vi "Header Footer Transform Header Footer [ ].vi"(7 "Header or Footer [ ]":T11[](array[typedef]), 11 "error in (no error)":errorcluster) -> (8 "Header or Footer Complete Cluster":T1, 15 "error out":errorcluster)   [LabVIEW 2012]
doc: "Version 1.0\nDeveloped by Jean-Marc Simard\nCopyright © 2010, Exaprom Inc.\nAll rights reserved.\nLicense: BSD\n\nWith iTextSharp 4.1.6 (http://itextsharp.sourceforge.net)\nunder Mozilla Public License Version 1.1\n(http://www.mozilla.org/MPL/MPL-1.1.html)"
uses:
  Controls/Header Footer cluster.ctl
  Controls/Header Footer Type.ctl
  Controls/Header footer horiz alignment.ctl
  Controls/Cell Vertical alignment.ctl
  Controls/Page number.ctl
  Controls/Font cluster.ctl
  Controls/Font size.ctl
  Controls/Font color.ctl
  C:/Users/MaxCorp/Documents/TopPerm - Base/DLL/itextsharp.dll
  DLL/itextsharp.dll
  Controls/Header Footer Line.ctl
  Controls/Header Footer Complete Cluster.ctl
  Controls/Header Footer Cluster with references.ctl
panel:
  # "X"
  # "Y"
  # "X"
  # "Y"
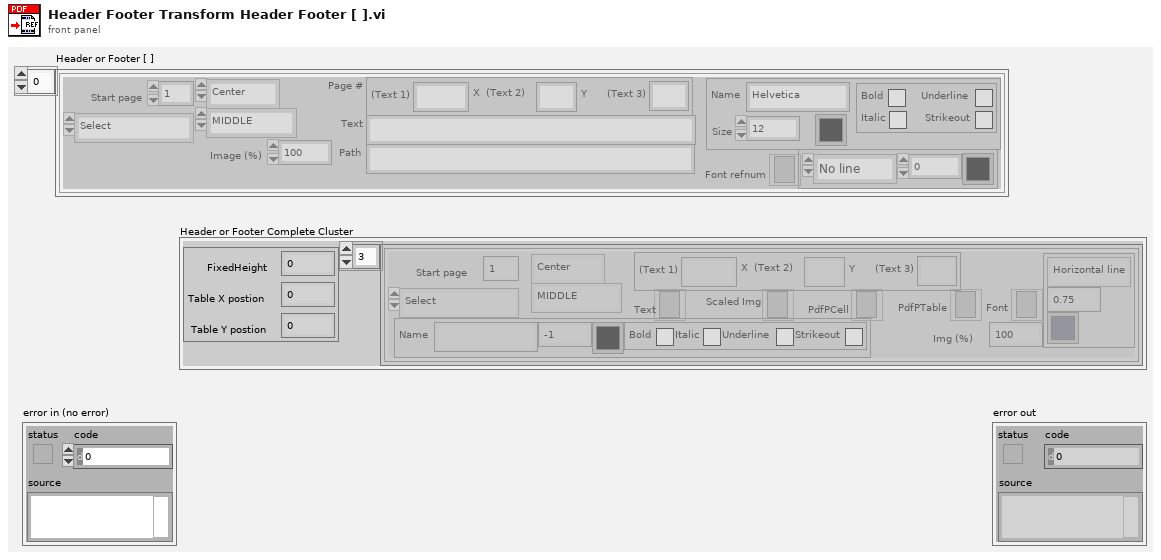
[diagram p1: front panel]
types:
  T1 = typedef "Header Footer Complete Cluster.ctl" = cluster{"Table position":cluster{"FixedHeight":dbl, "Table X postion":dbl, "Table Y postion":dbl}, "Header Footer Cluster with references [ ]":T2[]}
  T2 = typedef "Header Footer Cluster with references.ctl" = cluster{"Start page":i32, "Type":T3, "Alignment":T4, "Vertical Alignement":T5, "Page #":T6, "Text":refnum<k24>, "Scaled Img":refnum<k24>, "PdfPCell":refnum<k24>, "PdfPTable":refnum<k24>, "Font Cluster":T7, "Font ":refnum<k24>, "Img (%)":sgl, "Line":cluster{"Line":T10, "Thickness (points)":sgl, "Colour":T9}}
  T3 = typedef "Header Footer Type.ctl" = enum16{"Select", "Text", "Text + hyperlink", "Page number", "Image", "Image + hyperlink"}
  T4 = typedef "Header footer horiz alignment.ctl" = enum16{"Left", "Center", "Right"}
  T5 = typedef "Cell Vertical alignment.ctl" = enum16{"TOP", "MIDDLE", "BOTTOM"}
  T6 = typedef "Page number.ctl" = cluster{"Text 1":string, "Text 2":string, "Text 3":string}
  T7 = typedef "Font cluster.ctl" = cluster{"Name":string, "Size":T8, "Color":T9, "Style":cluster{"Bold":bool, "Italic":bool, "Underline":bool, "Strikeout":bool}}
  T8 = typedef "Font size.ctl" = sgl
  T9 = typedef "Font color.ctl" = u32
  T10 = typedef "Header Footer Line.ctl" = enum16{"No line", "Horizontal line"}
  T11 = typedef "Header Footer cluster.ctl" = cluster{"Start page":i32, "Type":T3, "Alignment":T4, "Vertical Alignement":T5, "Image (%)":sgl, "Page #":T6, "Text":string, "Path":string, "Font":T7, "Font refnum":refnum<k24>, "Line":cluster{"Line":T10, "Thickness (points)":sgl, "Colour":T9}}
  T12 = cluster{"FixedHeight":dbl, "Table X postion":dbl, "Table Y postion":dbl}
  T13 = cluster{"Line":T10, "Thickness (points)":sgl, "Colour":T9}
  T14 = cluster{"Table position":cluster{"FixedHeight":dbl, "Table X postion":dbl, "Table Y postion":dbl}, "Header Footer Cluster with references [ ]":T2[]}
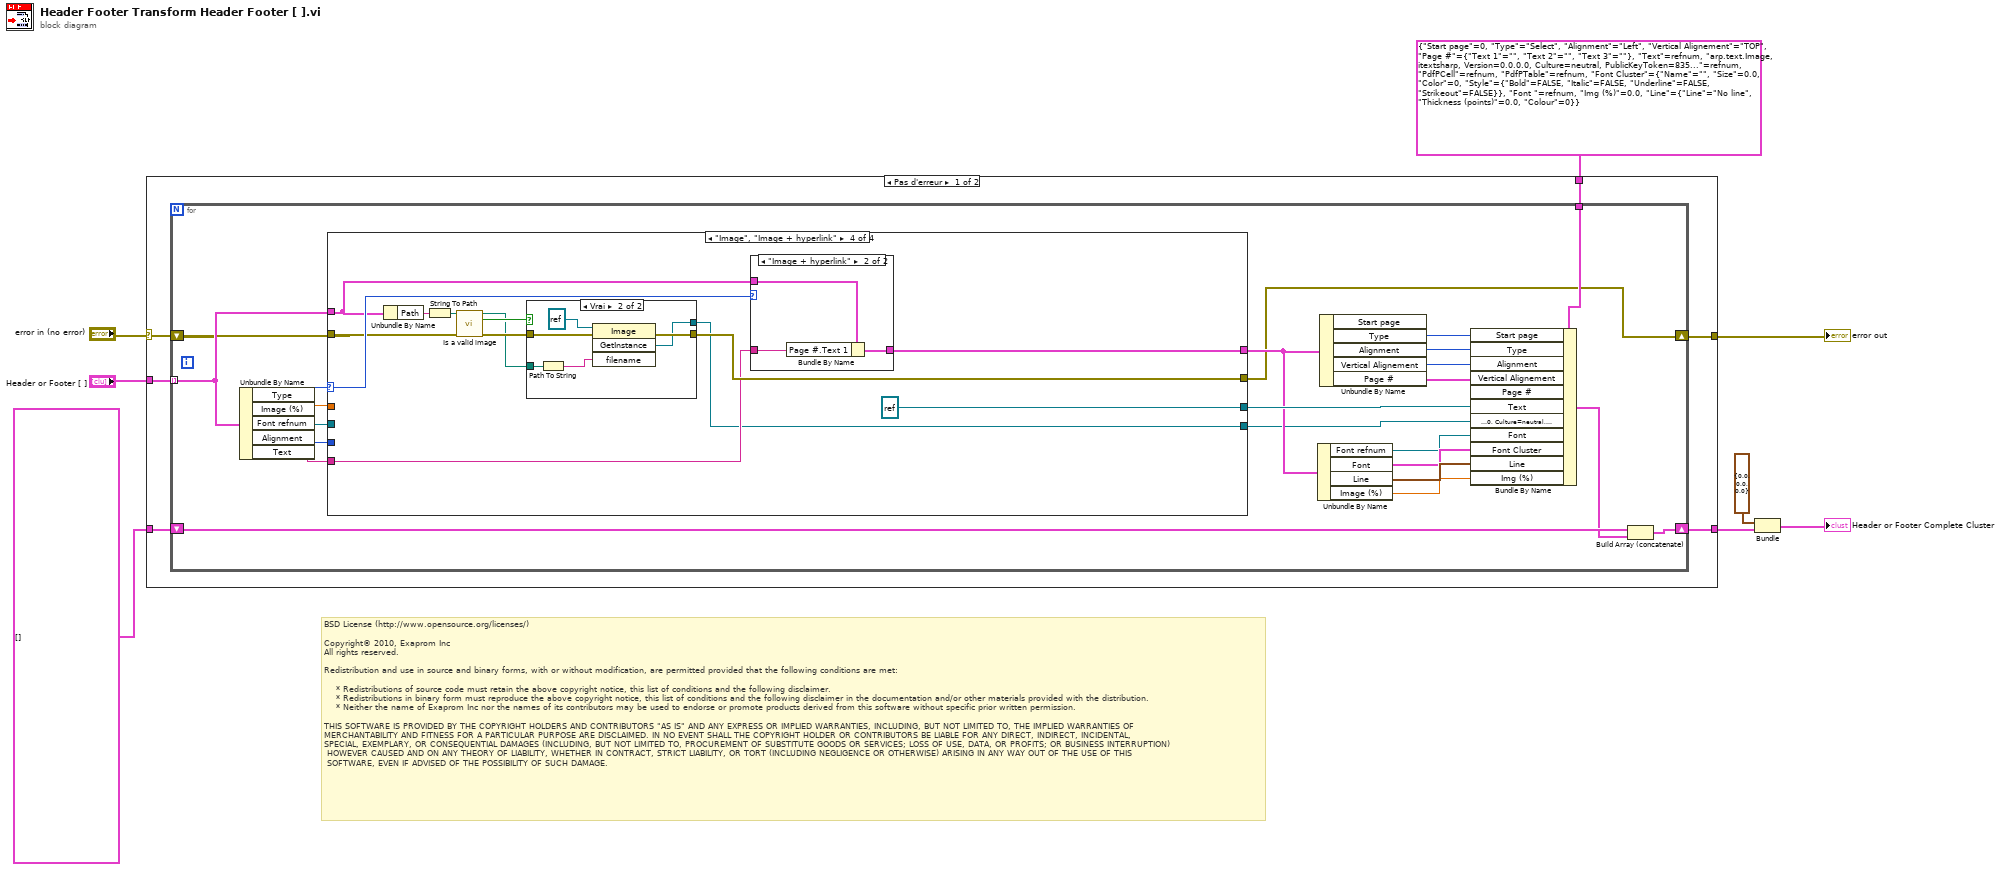
[diagram p0: block diagram]
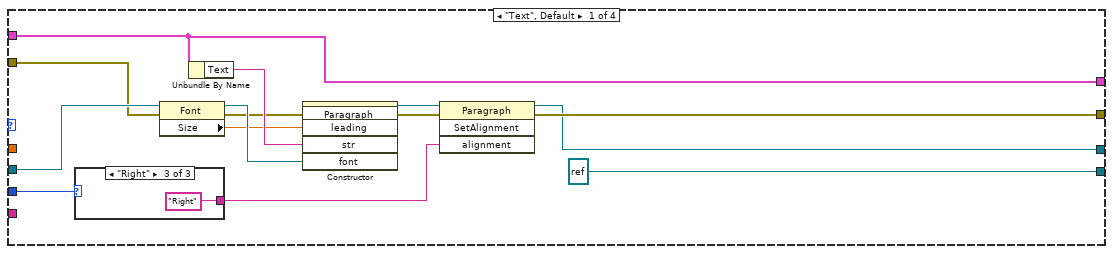
[diagram p2: hidden frame]
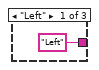
[diagram p3: hidden frame]
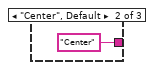
[diagram p4: hidden frame]
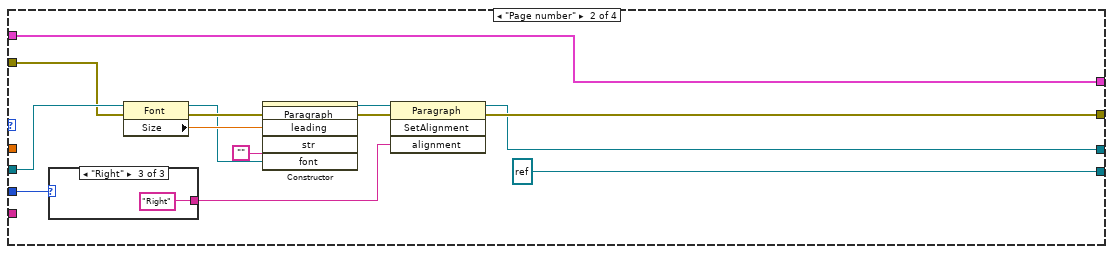
[diagram p5: hidden frame]
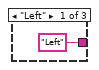
[diagram p6: hidden frame]
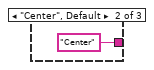
[diagram p7: hidden frame]
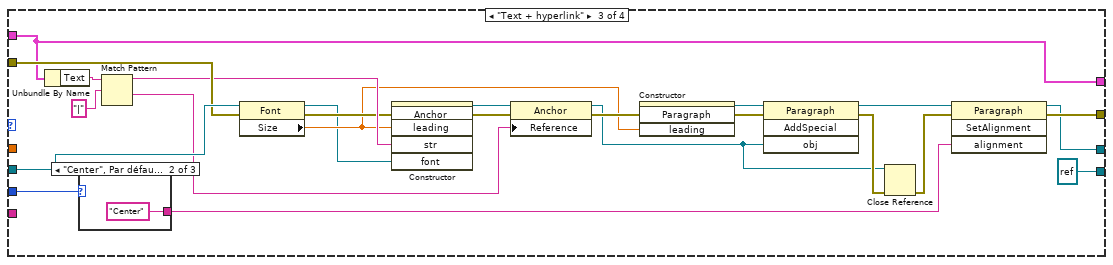
[diagram p8: hidden frame]
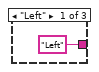
[diagram p9: hidden frame]
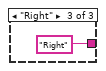
[diagram p10: hidden frame]
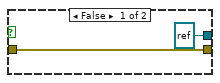
[diagram p11: hidden frame]
diagram:
  # "BSD License (http://www.opensource.org/licenses/)\n\nCopyright© 2010, Exaprom Inc\nAll rights reserved.\n\nRedistribution and use in source and binary forms, with or without modification, are permitted provided that the following conditions are met:\n\n    * Redistributions of source code must retain the above copyright notice, this list of conditions and the following disclaimer.\n    * Redistributions in binary form must reproduce the above copyright notice, this list of conditions and the following disclaimer in the documentation and/or other materials provided with the distribution.\n    * Neither the name of Exaprom Inc nor the names of its contributors may be used to endorse or promote products derived from this software without specific prior written permission.\n\nTHIS SOFTWARE IS PROVIDED BY THE COPYRIGHT HOLDERS AND CONTRIBUTORS \"AS IS\" AND ANY EXPRESS OR IMPLIED WARRANTIES, INCLUDING, BUT NOT LIMITED TO, THE IMPLIED WARRANTIES OF \nMERCHANTABILITY AND FITNESS FOR A PARTICULAR PURPOSE ARE DISCLAIMED. IN NO EVENT SHALL THE COPYRIGHT HOLDER OR CONTRIBUTORS BE LIABLE FOR ANY DIRECT, INDIRECT, INCIDENTAL,\nSPECIAL, EXEMPLARY, OR CONSEQUENTIAL DAMAGES (INCLUDING, BUT NOT LIMITED TO, PROCUREMENT OF SUBSTITUTE GOODS OR SERVICES; LOSS OF USE, DATA, OR PROFITS; OR BUSINESS INTERRUPTION)\n HOWEVER CAUSED AND ON ANY THEORY OF LIABILITY, WHETHER IN CONTRACT, STRICT LIABILITY, OR TORT (INCLUDING NEGLIGENCE OR OTHERWISE) ARISING IN ANY WAY OUT OF THE USE OF THIS\n SOFTWARE, EVEN IF ADVISED OF THE POSSIBILITY OF SUCH DAMAGE."
  n1 = case shown="Pas d'erreur" "error in (no error)" {
    selector: "error in (no error)" -> [w10 w126]
    tunnel: "Header or Footer [ ]" -> [w9 _]
    tunnel: [w14 w126] -> w8
    tunnel: T2 {"Start page"=0, "Type"=enum."Select", "Alignment"=enum."Left", "Vertical Alignement"=enum."TOP", "Page #"={"Text 1"="", "Text 2"="", "Text 3"=""}, "Text"=refnum, "Scaled Img"=refnum, "PdfPCell"=refnum, "PdfPTable"=refnum, "Font Cluster"={"Name"="", "Size"=0.0, "Color"=0, "Style"={"Bold"=FALSE, "Italic"=FALSE, "Underline"=FALSE, "Strikeout"=FALSE}}, "Font "=refnum, "Img (%)"=0.0, "Line"={"Line"=enum."No line", "Thickness (points)"=0.0, "Colour"=0}} ("Header Footer Cluster with references") -> [w13 _]
    tunnel: T2[] [] ("Header Footer Cluster with references [ ]") -> [w12 w125]
    tunnel: [w11 w125] -> w3
    frame No Error {
      n2 = for {
        tunnel: w9 -> [w24] mode=indexing
        tunnel: w13 -> [w33]
        shift-right: [w26] -> w11
        shift-left: w12 -> [w25]
        shift-right: [w19] -> w14
        shift-left: w10 -> [w22]
        n3 = Unbundle By Name(w24) -> ("Type"=w35:T3, "Image (%)"=w36:sgl, "Font refnum"=w38:refnum<k24>, "Alignment"=w37:T4, "Text"=w34:string)
        n4 = case shown="\"Image\", \"Image + hyperlink\"" w35 {
          selector: w35 -> [_ _ _ w110]
          tunnel: w24 -> [w47 w64 w91 w104]
          tunnel: w38 -> [w52 w69 w96 _]
          tunnel: w37 -> [w51 w68 w95 _]
          tunnel: w36 -> [_ _ _ _]
          tunnel: w34 -> [_ _ _ w108]
          tunnel: w22 -> [w50 w67 w94 w101]
          tunnel: [w46 w63 w90 refnum<k24> refnum ("new reference")] -> w27
          tunnel: [refnum<k24> refnum ("GetInstanceImage OUT") refnum<k24> refnum ("GetInstanceImage OUT") refnum<k24> refnum ("GetInstanceImage OUT") w107] -> w21
          tunnel: [w49 w66 w92 w111] -> w19
          tunnel: [w47 w64 w91 w109] -> w23
          frame "Text", Default {
            n5 = case shown="\"Right\"" w51 {
              tunnel: ["Left" "Center" "Right"] -> w43
              frame "Left" {
              }
              frame "Center", Default {
              }
              frame "Right" {
              }
            }
            n6 = property class="Font"(reference=w52, error in=w50) -> (reference out=w42:refnum<k24>, error out=w39:errorcluster, "Size"=w41:sgl)
            n7 = Unbundle By Name(w47) -> ("Text"=w45:string)
            n8 = constructor class="Paragraph"(error in=w39, "leading"=w41, "str"=w45, "font"=w42) -> (reference out=w44:refnum<k24>, error out=w40:errorcluster)  [unwired: 2 in, 4 out]
            n9 = invoke class="Paragraph" method="SetAlignment"(reference=w44, error in=w40, "alignment"=w43) -> (reference out=w46:refnum<k24>, error out=w49:errorcluster)  [unwired: 1 in, 2 out]
          }
          frame "Page number" {
            n10 = case shown="\"Right\"" w68 {
              tunnel: ["Left" "Center" "Right"] -> w60
              frame "Left" {
              }
              frame "Center", Default {
              }
              frame "Right" {
              }
            }
            n11 = property class="Font"(reference=w69, error in=w67) -> (reference out=w57:refnum<k24>, error out=w59:errorcluster, "Size"=w58:sgl)
            n12 = constructor class="Paragraph"(error in=w59, "leading"=w58, "str"="", "font"=w57) -> (reference out=w61:refnum<k24>, error out=w56:errorcluster)  [unwired: 2 in, 4 out]
            n13 = invoke class="Paragraph" method="SetAlignment"(reference=w61, error in=w56, "alignment"=w60) -> (reference out=w63:refnum<k24>, error out=w66:errorcluster)  [unwired: 1 in, 2 out]
          }
          frame "Text + hyperlink" {
            n14 = Unbundle By Name(w91) -> ("Text"=w86:string)
            n15 = case shown="\"Center\", Par défaut" w95 {
              tunnel: ["Left" "Center" "Right"] -> w89
              frame "Left" {
              }
              frame "Center", Default {
              }
              frame "Right" {
              }
            }
            n16 = Match Pattern(string=w86, regular expression="|") -> (before substring=w77:string, after substring=w84:string)  [unwired: 3 out]
            n17 = property class="Font"(reference=w96, error in=w94) -> (reference out=w73:refnum<k24>, error out=w75:errorcluster, "Size"=w74:sgl)
            n18 = constructor class="Anchor"(error in=w75, "leading"=w74, "str"=w77, "font"=w73) -> (reference out=w87:refnum<k24>, error out=w76:errorcluster)  [unwired: 2 in, 4 out]
            n19 = property class="Anchor"(reference=w87, error in=w76, "Reference"=w84) -> (reference out=w78:refnum<k24>, error out=w88:errorcluster)
            n20 = constructor class="Paragraph"(error in=w88, "leading"=w74) -> (reference out=w81:refnum<k24>, error out=w82:errorcluster)  [unwired: 2 in, 2 out]
            n21 = invoke class="Paragraph" method="AddSpecial"(reference=w81, error in=w82, "obj"=w78) -> (reference out=w83:refnum<k24>, error out=w80:errorcluster)  [unwired: 1 in, 2 out]
            n22 = Close Reference(reference=w78, error in (no error)=w80) -> (error out=w79:errorcluster)
            n23 = invoke class="Paragraph" method="SetAlignment"(reference=w83, error in=w79, "alignment"=w89) -> (reference out=w90:refnum<k24>, error out=w92:errorcluster)  [unwired: 1 in, 2 out]
          }
          frame "Image", "Image + hyperlink" {
            n24 = Unbundle By Name(w104) -> ("Path"=w105:string)
            n25 = String To Path(string=w105) -> (path=w106:path)
            n26 = call "Is a valid image.vi"("Image path"=w106, "error in (no error)"=w101) -> ("dup path"=w100:path, "Valid Image?"=w103:bool, "error out"=w102:errorcluster)  [unwired: 11 out]
            n27 = case shown="Vrai" w103 {
              tunnel: w100 -> [_ w119]
              tunnel: [w114 w118] -> w111
              tunnel: [refnum<k24> refnum ("GetInstance") w117] -> w107
              tunnel: w102 -> [w114 w116]
              frame False {
              }
              frame True {
                n28 = Path To String(path=w119) -> (string=w115:string)
                n29 = invoke class="Image" method="GetInstance"(reference=refnum<k24> refnum ("image"), error in=w116, "filename"=w115) -> (error out=w118:errorcluster, "GetInstance"=w117:refnum<k24>)  [unwired: 1 in, 2 out]
              }
            }
            n30 = case shown="\"Image + hyperlink\"" w110 {
              tunnel: [w121 w123] -> w109
              tunnel: w104 -> [w121 w124]
              tunnel: w108 -> [_ w122]
              frame "Select", Default {
              }
              frame "Image + hyperlink" {
                n31 = Bundle By Name(cluster=w124, "Page #.Text 1"=w122) -> (w123:T11)
              }
            }
          }
        }
        n32 = Unbundle By Name(w23) -> ("Font refnum"=w16:refnum<k24>, "Font"=w17:T7, "Line"=w18:T13, "Image (%)"=w15:sgl)
        n33 = Unbundle By Name(w23) -> ("Start page"=w32:i32, "Type"=w31:T3, "Alignment"=w30:T4, "Vertical Alignement"=w29:T5, "Page #"=w28:T6)
        n34 = Bundle By Name(cluster=w33, "Start page"=w32, "Type"=w31, "Alignment"=w30, "Vertical Alignement"=w29, "Page #"=w28, "Text"=w27, "Scaled Img"=w21, "Font"=w16, "Font Cluster"=w17, "Line"=w18, "Img (%)"=w15) -> (w20:T2)
        n35 = Build Array (concatenate)(w25, w20) -> (w26:T2[])
      }
    }
    frame Error {
    }
  }
  "error out" <- w8
  n36 = Bundle("Table position"=T12 {"FixedHeight"=0.0, "Table X postion"=0.0, "Table Y postion"=0.0}, "Header Footer Cluster with references [ ]"=w3) -> (→"Header or Footer Complete Cluster":T14)  [unwired: 1 out]
